vi "VI Main 1.1.vi"() -> ()   [LabVIEW 2014]
uses:
  <vilib>/Analysis/NI_AALPro.lvlib
panel:
  in  "clear graph at start":bool
  in  "clear graph":bool
  out "Elapsed Time":dbl format="%<%H:%M:%S>t"
  out "Measuring!":bool
  out "Current Interval":i32
  out "Benchmark (s)":dbl format="%.2g"
  out "Start time":timestamp
  in  "STOP acq":bool
  in  "# of Intervals":i32=1 min=2 step=1
  in  "Interval (s)":dbl=2.0 min=3.0 step=1.0
  in  "Quick Acq":bool
  in  "Multi Acq":bool
  in  "Reset":bool
  in  "Single Acq":bool
  in  "stop":bool
  out "intercept":dbl format="%_4g"
  out "Waveform Chart":dbl(graph)=1498.7145698358406
  out "Res. (ohm)":dbl format="%#.5g"
  out "XY Graph":cluster{dbl[], "Best Linear Fit":dbl[]}[](graph)=[{[0.0, 0.263, 0.5265, 0.7895, 1.0525, 1.3159999999999998, 1.579, 1.8419999999999999, 2.1054999999999997, 2.3685, 2.6315, 2.8945, 3.158, 3.421, 3.6839999999999997, 3.9475, 4.2105, 4.4735, 4.737, 5.0], "Best Linear Fit"=[8.396237e-09, 0.00017563, 0.0003515037, 0.0005267256, 0.0007024271000000001, 0.0008784534, 0.0010530580000000002, 0.001229876, 0.0014040270000000002, 0.0015802980000000002, 0.0017562010000000002, 0.001931084, 0.002107921, 0.002282894, 0.002458404, 0.002635005, 0.0028083120000000003, 0.0029850220000000004, 0.0031614950000000003, 0.003335616]}, {[0.0, 0.263, 0.5265, 0.7895, 1.0525, 1.3159999999999998, 1.579, 1.8419999999999999, 2.1054999999999997, 2.3685, 2.6315, 2.8945, 3.158, 3.421, 3.6839999999999997, 3.9475, 4.2105, 4.4735, 4.737, 5.0], "Best Linear Fit"=[8.582660926425292e-08, 0.00017557123354217628, 0.0003513902629217288, 0.0005268756698546408, 0.0007023610767875529, 0.0008781801061671053, 0.0010536655131000174, 0.0012291509200329294, 0.0014049699494124818, 0.001580455356345394, 0.0017559407632783061, 0.001931426170211218, 0.0021072451995907708, 0.0022827306065236826, 0.0024582160134565944, 0.0026340350428361472, 0.002809520449769059, 0.002985005856701971, 0.0031608248860815237, 0.003336310293014436]}]
  in  "Sense range":i32(slide)
  in  "Stop (V)":dbl=5.0 format="%.4f"
  in  "Source compliance (A)":dbl=0.01 format="%.4f"
  in  "Direction":i32(slide)
  in  "Ranging":i32(slide)
  in  "Start (V)":dbl step=1.0 format="%.4p"
  in  "# of points to acquire":i32=20 min=1 max=2500 step=1
  in  "Speed":i32(slide)=2
  out "status":i32 format="%.0x"
  in  "resource name 2":string="GPIB4::24::INSTR"
  in  "resource name":string="ASRL4::INSTR"
  out "Qrun":bool
  out "Mrun":bool
  out "Srun":bool
  # ">"
  # "by L.Andrzejewski\nlandrzej@uottawa.ca"
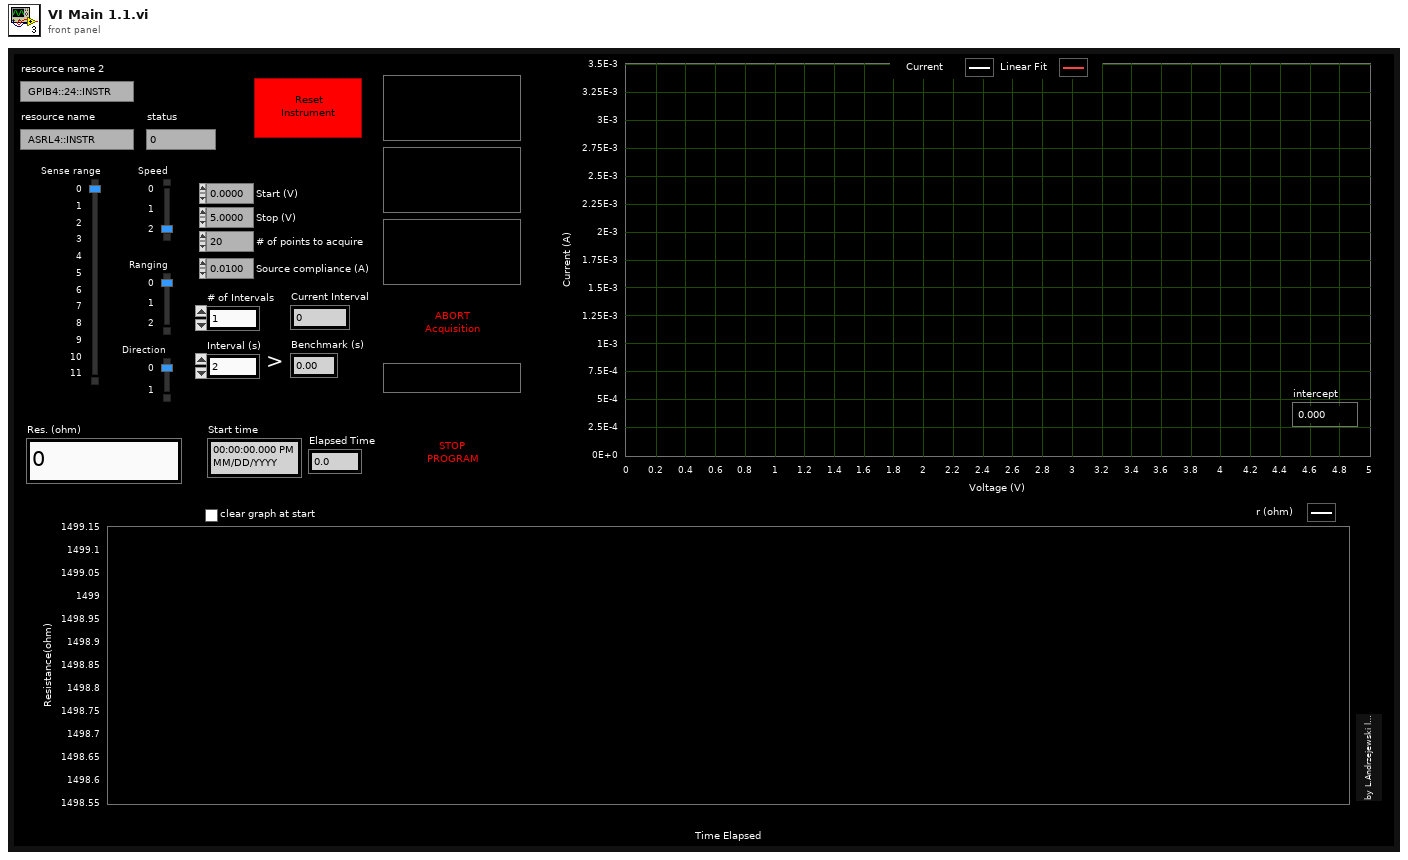
[diagram p1: front panel]
types:
  T1 = enum8{"Enabled", "Disabled", "Disabled and Grayed Out"}
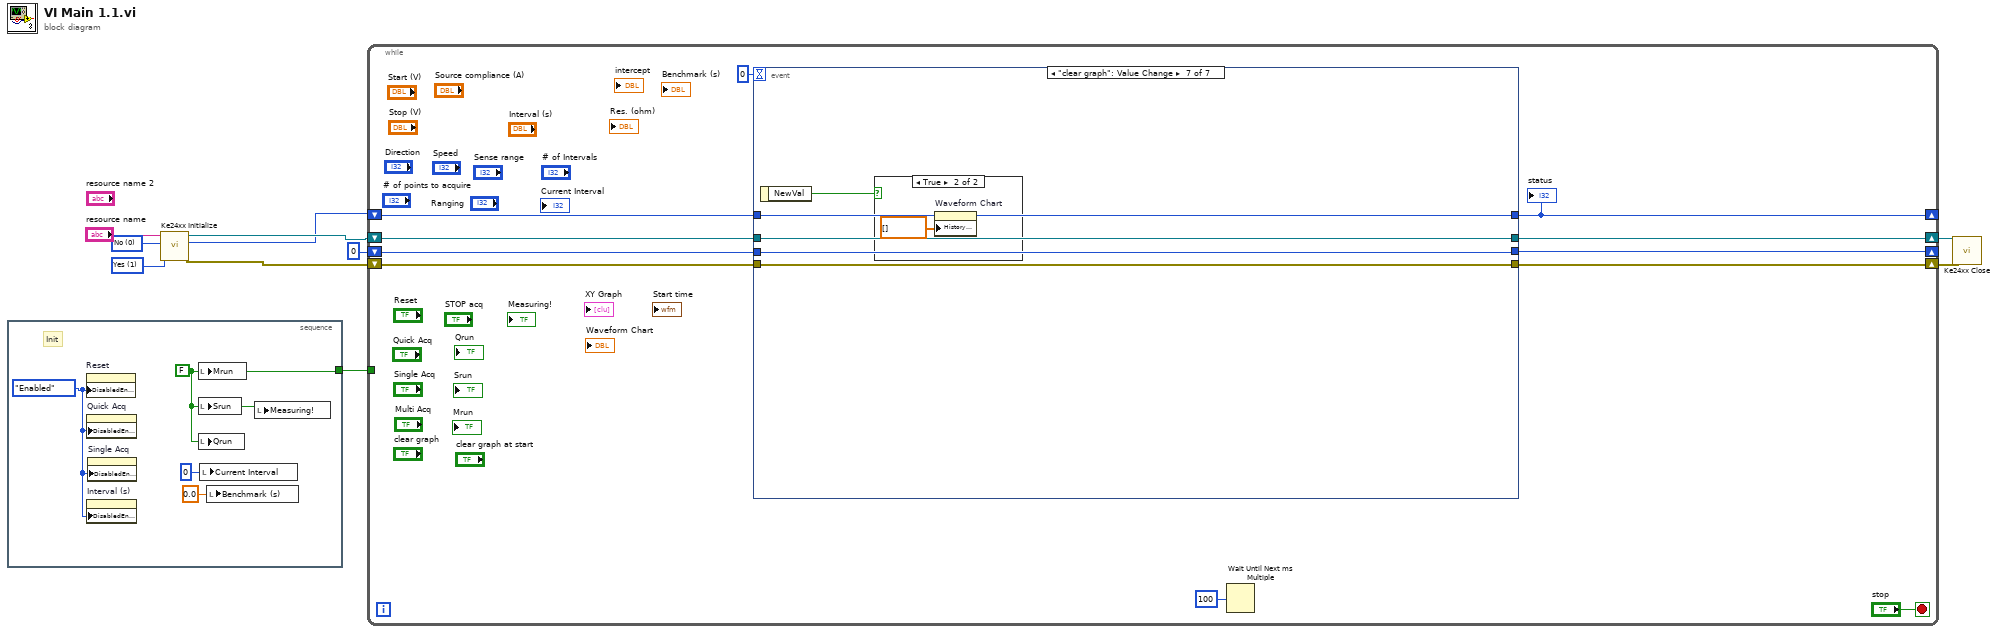
[diagram p0: block diagram]
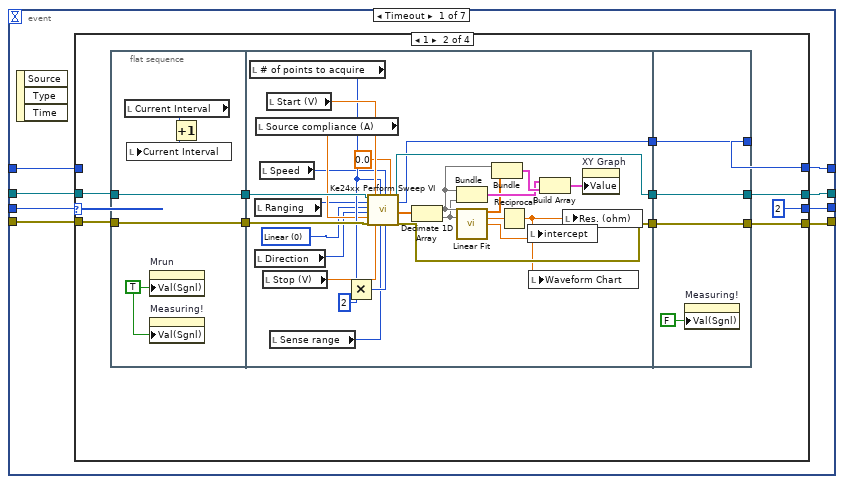
[diagram p2: hidden frame]
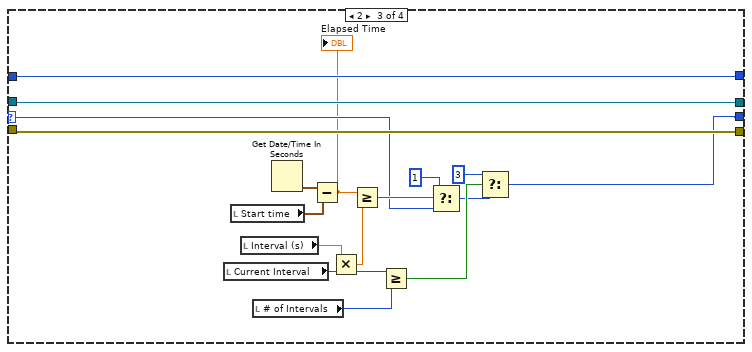
[diagram p4: hidden frame]
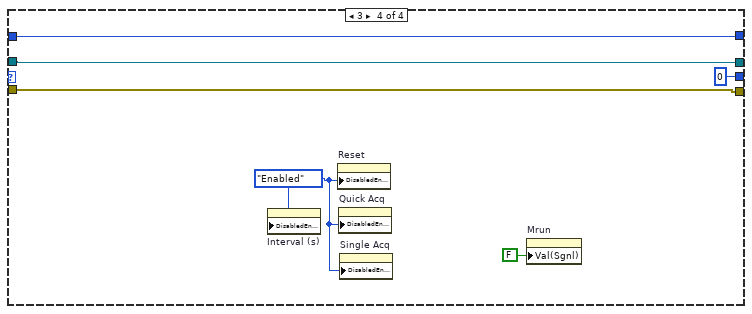
[diagram p5: hidden frame]
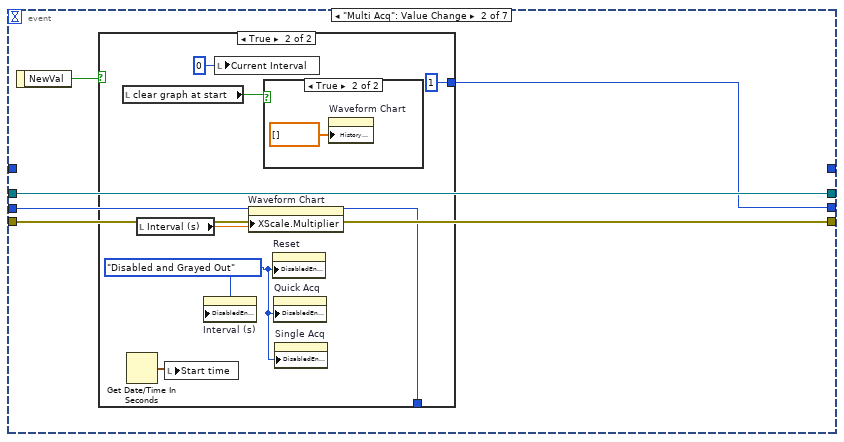
[diagram p6: hidden frame]
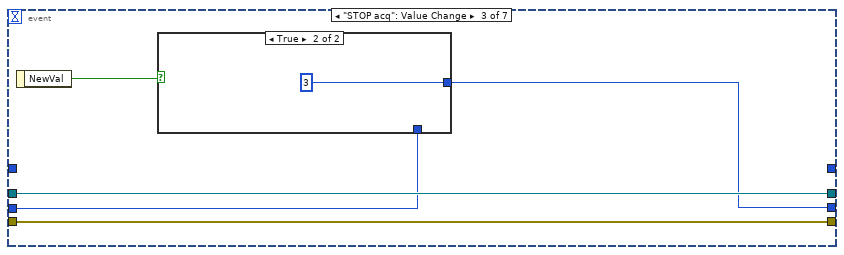
[diagram p9: hidden frame]
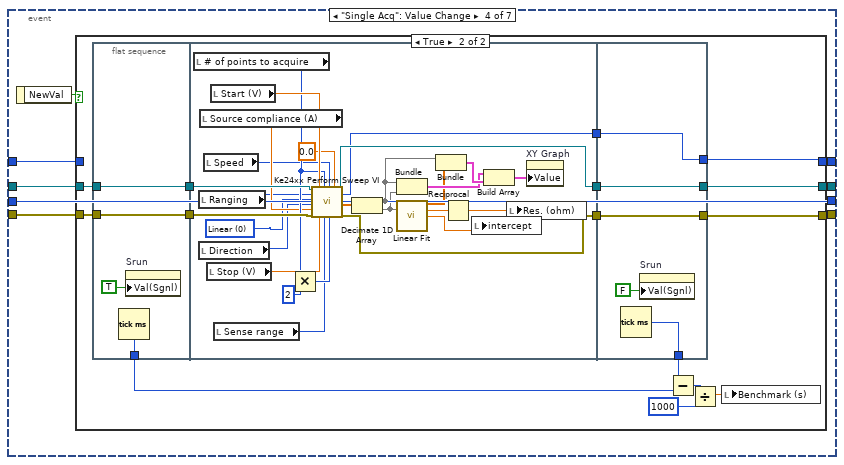
[diagram p11: hidden frame]
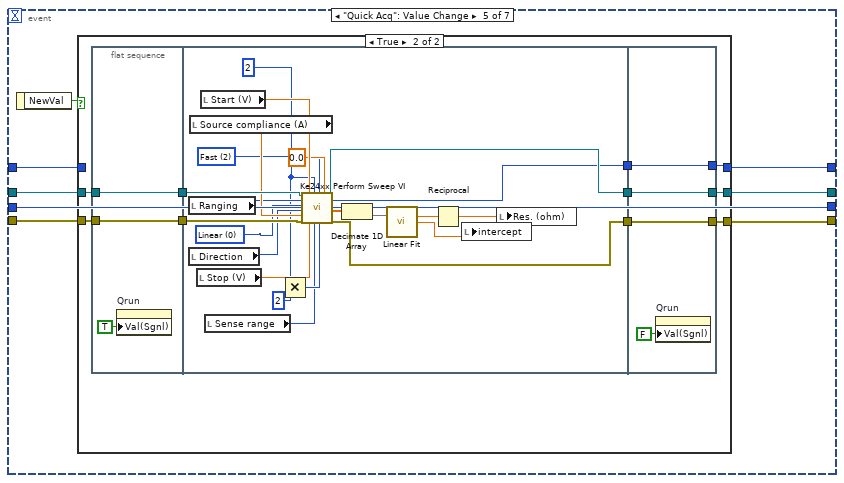
[diagram p13: hidden frame]
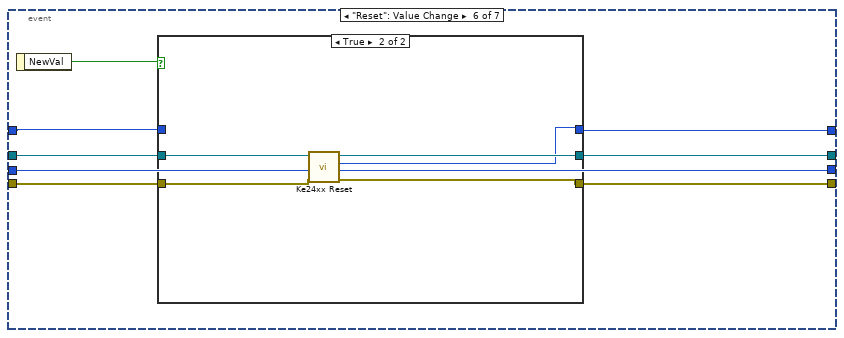
[diagram p15: hidden frame]
diagram:
  w9 = u16 1 items=["Yes"=1, "No"=0] ("id query")
  w10 = u16 0 items=["Yes"=1, "No"=0] ("reset device")
  n1 = stacked-sequence {
    tunnel: [w12] -> w2
    frame #0 {
      w11 = T1."Enabled" ("Disabled")
      w12 = FALSE ("Mrun")
      # "Init"
      n2 = property on="Reset" class="Bool"("DisabledEnum"=w11) -> ()  [unwired: 2 in, 2 out]
      n3 = property on="Quick Acq" class="Bool"("DisabledEnum"=w11) -> ()  [unwired: 2 in, 2 out]
      n4 = property on="Interval (s)" class="DigNum (strict)"("DisabledEnum"=w11) -> ()  [unwired: 2 in, 2 out]
      n5 = property on="Single Acq" class="Bool"("DisabledEnum"=w11) -> ()  [unwired: 2 in, 2 out]
      n6 = local write "Mrun"(w12) -> ()
      n7 = local write "Srun"(w12) -> ()
      n8 = local write "Qrun"(w12) -> ()
      n9 = local write "Current Interval"(0 ("Current Interval")) -> ()
      n10 = local write "Benchmark (s)"(0.0 ("Benchmark (s)")) -> ()
      n11 = local write "Measuring!"(w12) -> ()
    }
  }
  n12 = call <instrlib>:"Ke24xx Initialize.vi"("reset device"=w10, "id query"=w9, "resource name"="resource name") -> ("error out"=w3:errorcluster, "status"=w4:i32, "instrument handle out"=w5:refnum<visa-resource-name>)  [unwired: 6 in]
  n13 = while {
    shift-right: [w20] -> w7
    shift-left: w5 -> [w22]
    shift-right: [w19] -> w6
    shift-left: w3 -> [w21]
    shift-right: [w17] -> _
    shift-left: w4 -> [w18]
    tunnel: w2 -> [_]
    shift-right: [w15] -> _
    shift-left: 0 -> [w16]
    stop <- "stop" stop-if-true
    n14 = event shown="[6] \"clear graph\": Value Change" {
      selector: _ -> [_ _ _ _ _ _ _]
      dyn-events: _ -> [_ _ _ _ _ _ _]
      timeout: 0 -> [_ _ _ _ _ _ _]
      tunnel: [w29 w111 w124 w131 w193 w244 w259] -> w20
      tunnel: w22 -> [w32 w111 w124 w134 w196 w245 w259]
      tunnel: [w28 w110 w123 w132 w194 w243 w257] -> w19
      tunnel: w21 -> [w31 w110 w123 w133 w195 w242 w257]
      tunnel: w18 -> [w30 _ _ w130 w192 w247 w260]
      tunnel: [w26 _ _ w129 w191 w246 w260] -> w17
      tunnel: w16 -> [w33 w108 w121 w128 w190 w241 w258]
      tunnel: [w27 w109 w122 w128 w190 w241 w258] -> w15
      event Timeout {
        n15 = event-data() -> ()  [unwired: 1 in, 3 out]
        n16 = case shown="1" w33 {
          selector: w33 -> [w34 _ w90 _]
          tunnel: w32 -> [w36 w46 w99 w105]
          tunnel: w31 -> [w35 w45 w100 w103]
          tunnel: w30 -> [w37 _ w101 w106]
          tunnel: [w36 w44 w99 w105] -> w29
          tunnel: [w35 w43 w100 w103] -> w28
          tunnel: [w34 2 w87 0 ("t")] -> w27
          tunnel: [w37 w41 w101 w106] -> w26
          frame 0, Default {
          }
          frame 1 {
            n17 = flat-sequence {
              tunnel: w45 -> [w52]
              tunnel: w46 -> [w53]
              tunnel: [w53] -> w48
              tunnel: [w52] -> w47
              tunnel: w48 -> [w73]
              tunnel: w47 -> [w72]
              tunnel: [w71] -> w40
              tunnel: [w70] -> w39
              tunnel: [w55] -> w38
              tunnel: [w82] -> w41
              tunnel: [w83] -> w44
              tunnel: [w84] -> w43
              tunnel: w40 -> [w84]
              tunnel: w39 -> [w83]
              tunnel: w38 -> [w82]
              frame #0 {
                w49 = TRUE ("Value (Signaling)")
                n18 = local read "Current Interval"() -> (w50:i32)
                n19 = property on="Mrun" class="Bool (strict)"("Val(Sgnl)"=w49) -> ()  [unwired: 2 in, 2 out]
                n20 = property on="Measuring!" class="Bool (strict)"("Val(Sgnl)"=w49) -> ()  [unwired: 2 in, 2 out]
                n21 = Increment(x=w50) -> (x+1=w51:i32)
                n22 = local write "Current Interval"(w51) -> ()
              }
              frame #1 {
                w57 = 0 items=["Linear", "Logarithmic"] ("spacing")
                n23 = local read "# of points to acquire"() -> (w64:i32)
                n24 = local read "Ranging"() -> (w59:i32)
                n25 = local read "Direction"() -> (w58:i32)
                n26 = local read "Source compliance (A)"() -> (w61:dbl)
                n27 = local read "Speed"() -> (w60:i32)
                n28 = local read "Stop (V)"() -> (w66:dbl)
                n29 = local read "Start (V)"() -> (w67:dbl)
                n30 = local read "Sense range"() -> (w62:i32)
                n31 = Multiply(x=w64, y=2) -> (x*y=w63:i32)
                n32 = call <instrlib>:"Ke24xx Perform Sweep VI.vi"("instrument handle"=w73, "ranging"=w59, "spacing"=w57, "direction"=w58, "source compliance"=w61, "error in (no error)"=w72, "start"=w67, "stop"=w66, "number of points"=w64, "sense range"=w62, "speed"=w60, "size of reading"=w63, "source protection"=0.0) -> ("instrument handle out"=w70:refnum<visa-resource-name>, "status"=w55:i32, "out"=w74:dbl[], "error out"=w71:errorcluster)  [unwired: 3 in]
                n33 = Decimate 1D Array(w74) -> (w78:dbl[], w75:dbl[])
                n34 = Bundle(w78, w75) -> (w79:cluster{dbl[], dbl[]})  [unwired: 1 in]
                n35 = call <vilib>:"Linear Fit.vi"("Y"=w75, "X"=w78) -> ("Best Linear Fit"=w77:dbl[], "slope"=w76:dbl, "intercept"=w69:dbl)  [unwired: 9 in, 2 out]
                n36 = Bundle(w78, "Best Linear Fit"=w77) -> (w80:cluster{dbl[], "Best Linear Fit":dbl[]})  [unwired: 1 in]
                n37 = Reciprocal(x=w76) -> (1/x=w54:dbl)
                n38 = local write "intercept"(w69) -> ()
                n39 = local write "Waveform Chart"(w54) -> ()
                n40 = Build Array(w79, w80) -> (w68:cluster{dbl[], "Best Linear Fit":dbl[]}[])
                n41 = local write "Res. (ohm)"(w54) -> ()
                n42 = property on="XY Graph" class="XYGraph (strict)"("Value"=w68) -> ()  [unwired: 2 in, 2 out]
              }
              frame #2 {
                n43 = property on="Measuring!" class="Bool (strict)"("Val(Sgnl)"=FALSE ("Value (Signaling)")) -> ()  [unwired: 2 in, 2 out]
              }
            }
          }
          frame 2 {
            n44 = local read "Current Interval"() -> (w93:i32)
            n45 = local read "Start time"() -> (w97:timestamp)
            n46 = local read "Interval (s)"() -> (w96:dbl)
            n47 = local read "# of Intervals"() -> (w92:i32)
            n48 = Get Date/Time In Seconds() -> (seconds since 1Jan1904=w98:timestamp)
            n49 = Subtract(x=w98, y=w97) -> (x-y=w85:dbl)
            "Elapsed Time" <- w85
            n50 = Multiply(x=w96, y=w93) -> (x*y=w95:dbl)
            n51 = Greater Or Equal?(x=w85, y=w95) -> (x >= y?=w94:bool)
            n52 = Greater Or Equal?(x=w93, y=w92) -> (x >= y?=w89:bool)
            n53 = Select(t=1, s=w94, f=w90) -> (s? t:f=w88:i32)
            n54 = Select(t=3, s=w89, f=w88) -> (s? t:f=w87:i32)
          }
          frame 3 {
            w102 = T1."Enabled" ("Disabled")
            n55 = property on="Interval (s)" class="DigNum (strict)"("DisabledEnum"=w102) -> ()  [unwired: 2 in, 2 out]
            n56 = property on="Reset" class="Bool"("DisabledEnum"=w102) -> ()  [unwired: 2 in, 2 out]
            n57 = property on="Quick Acq" class="Bool"("DisabledEnum"=w102) -> ()  [unwired: 2 in, 2 out]
            n58 = property on="Single Acq" class="Bool"("DisabledEnum"=w102) -> ()  [unwired: 2 in, 2 out]
            n59 = property on="Mrun" class="Bool (strict)"("Val(Sgnl)"=FALSE ("Value (Signaling)")) -> ()  [unwired: 2 in, 2 out]
          }
        }
      }
      event "Multi Acq": Value Change {
        n60 = event-data() -> ("NewVal"=w112:bool)  [unwired: 1 in]
        n61 = case shown="True" w112 {
          tunnel: [w113 1] -> w109
          tunnel: w108 -> [w113 _]
          frame False {
          }
          frame True {
            w115 = T1."Disabled and Grayed Out" ("Disabled")
            n62 = local read "clear graph at start"() -> (w114:bool)
            n63 = Get Date/Time In Seconds() -> (seconds since 1Jan1904=w117:timestamp)
            n64 = local read "Interval (s)"() -> (w116:dbl)
            n65 = local write "Start time"(w117) -> ()
            n66 = property on="Interval (s)" class="DigNum (strict)"("DisabledEnum"=w115) -> ()  [unwired: 2 in, 2 out]
            n67 = local write "Current Interval"(0 ("Current Interval")) -> ()
            n68 = property on="Waveform Chart" class="WFChart (strict)"("XScale.Multiplier"=w116) -> ()  [unwired: 2 in, 2 out]
            n69 = case shown="True" w114 {
              frame False {
              }
              frame True {
                n70 = property on="Waveform Chart" class="WFChart (strict)"("History Data"=dbl[] []) -> ()  [unwired: 2 in, 2 out]
              }
            }
            n71 = property on="Reset" class="Bool"("DisabledEnum"=w115) -> ()  [unwired: 2 in, 2 out]
            n72 = property on="Quick Acq" class="Bool"("DisabledEnum"=w115) -> ()  [unwired: 2 in, 2 out]
            n73 = property on="Single Acq" class="Bool"("DisabledEnum"=w115) -> ()  [unwired: 2 in, 2 out]
          }
        }
      }
      event "STOP acq": Value Change {
        n74 = event-data() -> ("NewVal"=w125:bool)  [unwired: 1 in]
        n75 = case shown="True" w125 {
          tunnel: [w126 3] -> w122
          tunnel: w121 -> [w126 _]
          frame False {
          }
          frame True {
          }
        }
      }
      event "Single Acq": Value Change {
        n76 = event-data() -> ("NewVal"=w135:bool)  [unwired: 1 in]
        n77 = case shown="True" w135 {
          tunnel: w134 -> [w138 w153]
          tunnel: w133 -> [w137 w152]
          tunnel: [w137 w151] -> w132
          tunnel: [w138 w150] -> w131
          tunnel: [w136 w145] -> w129
          tunnel: w130 -> [w136 _]
          frame False {
          }
          frame True {
            n78 = flat-sequence {
              tunnel: w152 -> [w156]
              tunnel: w153 -> [w157]
              tunnel: [w157] -> w147
              tunnel: [w156] -> w146
              tunnel: [w154] -> w142
              tunnel: [w175] -> w149
              tunnel: [w174] -> w148
              tunnel: w147 -> [w177]
              tunnel: w146 -> [w176]
              tunnel: [w158] -> w144
              tunnel: [w188] -> w150
              tunnel: [w189] -> w151
              tunnel: w149 -> [w189]
              tunnel: w148 -> [w188]
              tunnel: [w187] -> w145
              tunnel: w144 -> [w187]
              tunnel: [w185] -> w143
              frame #0 {
                n79 = Tick Count (ms)() -> (millisecond timer value=w154:u32)
                n80 = property on="Srun" class="Bool (strict)"("Val(Sgnl)"=TRUE ("Value (Signaling)")) -> ()  [unwired: 2 in, 2 out]
              }
              frame #1 {
                w160 = 0 items=["Linear", "Logarithmic"] ("spacing")
                n81 = local read "# of points to acquire"() -> (w167:i32)
                n82 = local read "Ranging"() -> (w162:i32)
                n83 = local read "Direction"() -> (w161:i32)
                n84 = local read "Source compliance (A)"() -> (w164:dbl)
                n85 = local read "Speed"() -> (w163:i32)
                n86 = local read "Stop (V)"() -> (w169:dbl)
                n87 = local read "Start (V)"() -> (w170:dbl)
                n88 = local read "Sense range"() -> (w165:i32)
                n89 = Multiply(x=w167, y=2) -> (x*y=w166:i32)
                n90 = call <instrlib>:"Ke24xx Perform Sweep VI.vi"("instrument handle"=w177, "ranging"=w162, "spacing"=w160, "direction"=w161, "source compliance"=w164, "error in (no error)"=w176, "start"=w170, "stop"=w169, "number of points"=w167, "sense range"=w165, "speed"=w163, "size of reading"=w166, "source protection"=0.0) -> ("instrument handle out"=w174:refnum<visa-resource-name>, "status"=w158:i32, "out"=w178:dbl[], "error out"=w175:errorcluster)  [unwired: 3 in]
                n91 = Decimate 1D Array(w178) -> (w182:dbl[], w179:dbl[])
                n92 = Bundle(w182, w179) -> (w183:cluster{dbl[], dbl[]})  [unwired: 1 in]
                n93 = call <vilib>:"Linear Fit.vi"("Y"=w179, "X"=w182) -> ("Best Linear Fit"=w181:dbl[], "slope"=w180:dbl, "intercept"=w173:dbl)  [unwired: 9 in, 2 out]
                n94 = Bundle(w182, "Best Linear Fit"=w181) -> (w184:cluster{dbl[], "Best Linear Fit":dbl[]})  [unwired: 1 in]
                n95 = Reciprocal(x=w180) -> (1/x=w172:dbl)
                n96 = local write "intercept"(w173) -> ()
                n97 = Build Array(w183, w184) -> (w171:cluster{dbl[], "Best Linear Fit":dbl[]}[])
                n98 = local write "Res. (ohm)"(w172) -> ()
                n99 = property on="XY Graph" class="XYGraph (strict)"("Value"=w171) -> ()  [unwired: 2 in, 2 out]
              }
              frame #2 {
                n100 = Tick Count (ms)() -> (millisecond timer value=w185:u32)
                n101 = property on="Srun" class="Bool (strict)"("Val(Sgnl)"=FALSE ("Value (Signaling)")) -> ()  [unwired: 2 in, 2 out]
              }
            }
            n102 = Subtract(x=w143, y=w142) -> (x-y=w141:u32)
            n103 = Divide(x=w141, y=u32 1000) -> (x/y=w139:dbl)
            n104 = local write "Benchmark (s)"(w139) -> ()
          }
        }
      }
      event "Quick Acq": Value Change {
        n105 = event-data() -> ("NewVal"=w197:bool)  [unwired: 1 in]
        n106 = case shown="True" w197 {
          tunnel: w196 -> [w200 w210]
          tunnel: w195 -> [w199 w209]
          tunnel: [w199 w208] -> w194
          tunnel: [w200 w207] -> w193
          tunnel: [w198 w202] -> w191
          tunnel: w192 -> [w198 _]
          frame False {
          }
          frame True {
            n107 = flat-sequence {
              tunnel: w209 -> [w212]
              tunnel: w210 -> [w213]
              tunnel: [w213] -> w206
              tunnel: [w212] -> w205
              tunnel: w206 -> [w232]
              tunnel: w205 -> [w231]
              tunnel: [w230] -> w204
              tunnel: [w229] -> w203
              tunnel: [w214] -> w201
              tunnel: [w239] -> w207
              tunnel: [w240] -> w208
              tunnel: w204 -> [w240]
              tunnel: w203 -> [w239]
              tunnel: [w237] -> w202
              tunnel: w201 -> [w237]
              frame #0 {
                n108 = property on="Qrun" class="Bool (strict)"("Val(Sgnl)"=TRUE ("Qrun")) -> ()  [unwired: 2 in, 2 out]
              }
              frame #1 {
                w215 = 2 items=["Slow", "Medium", "Fast"] ("speed")
                w216 = 2 ("x")
                w218 = 0 items=["Linear", "Logarithmic"] ("spacing")
                n109 = local read "Ranging"() -> (w220:i32)
                n110 = local read "Direction"() -> (w219:i32)
                n111 = local read "Source compliance (A)"() -> (w221:dbl)
                n112 = local read "Stop (V)"() -> (w225:dbl)
                n113 = local read "Start (V)"() -> (w226:dbl)
                n114 = local read "Sense range"() -> (w222:i32)
                n115 = Multiply(x=w216, y=2) -> (x*y=w223:i32)
                n116 = call <instrlib>:"Ke24xx Perform Sweep VI.vi"("instrument handle"=w232, "ranging"=w220, "spacing"=w218, "direction"=w219, "source compliance"=w221, "error in (no error)"=w231, "start"=w226, "stop"=w225, "number of points"=w216, "sense range"=w222, "speed"=w215, "size of reading"=w223, "source protection"=0.0) -> ("instrument handle out"=w229:refnum<visa-resource-name>, "status"=w214:i32, "out"=w233:dbl[], "error out"=w230:errorcluster)  [unwired: 3 in]
                n117 = Decimate 1D Array(w233) -> (w236:dbl[], w234:dbl[])
                n118 = call <vilib>:"Linear Fit.vi"("Y"=w234, "X"=w236) -> ("slope"=w235:dbl, "intercept"=w228:dbl)  [unwired: 9 in, 3 out]
                n119 = Reciprocal(x=w235) -> (1/x=w227:dbl)
                n120 = local write "intercept"(w228) -> ()
                n121 = local write "Res. (ohm)"(w227) -> ()
              }
              frame #2 {
                n122 = property on="Qrun" class="Bool (strict)"("Val(Sgnl)"=FALSE ("Qrun")) -> ()  [unwired: 2 in, 2 out]
              }
            }
          }
        }
      }
      event "Reset": Value Change {
        n123 = event-data() -> ("NewVal"=w248:bool)  [unwired: 1 in]
        n124 = case shown="True" w248 {
          tunnel: [w251 w252] -> w246
          tunnel: w247 -> [w251 _]
          tunnel: w245 -> [w250 w256]
          tunnel: [w250 w255] -> w244
          tunnel: [w249 w253] -> w243
          tunnel: w242 -> [w249 w254]
          frame False {
          }
          frame True {
            n125 = call <instrlib>:"Ke24xx Reset.vi"("error in (no error)"=w254, "instrument handle"=w256) -> ("error out"=w253:errorcluster, "status"=w252:i32, "instrument handle out"=w255:refnum<visa-resource-name>)  [unwired: 7 in]
          }
        }
      }
      event "clear graph": Value Change {
        n126 = event-data() -> ("NewVal"=w261:bool)  [unwired: 1 in]
        n127 = case shown="True" w261 {
          frame False {
          }
          frame True {
            n128 = property on="Waveform Chart" class="WFChart (strict)"("History Data"=dbl[] []) -> ()  [unwired: 2 in, 2 out]
          }
        }
      }
    }
    "status" <- w17
    n129 = Wait Until Next ms Multiple(millisecond multiple=u32 100) -> ()  [unwired: 1 out]
  }
  n130 = call <instrlib>:"Ke24xx Close.vi"("error in (no error)"=w6, "instrument handle"=w7) -> ()  [unwired: 8 in, 2 out]
